vi "GT Pvt Table.vi"(0 "cardNum":i16, 1 "pPos":dbl, 5 "tableId":i16, 7 "count":i32, 9 "pTime":dbl, 11 "error in (no error)":errorcluster caption="错误输入（无错误）", 12 "pVel":dbl) -> (3 "pPos out":dbl, 4 "function return":i16, 10 "pTime out":dbl, 14 "pVel out":dbl, 15 "error out":errorcluster caption="错误输出")   [LabVIEW 2014, in "gts.lvlib"]
doc: "GT_API GT_PvtTable(short cardNum,short tableId,long count,double *pTime,double *pPos,double *pVel);"
uses:
  gts.lvlib
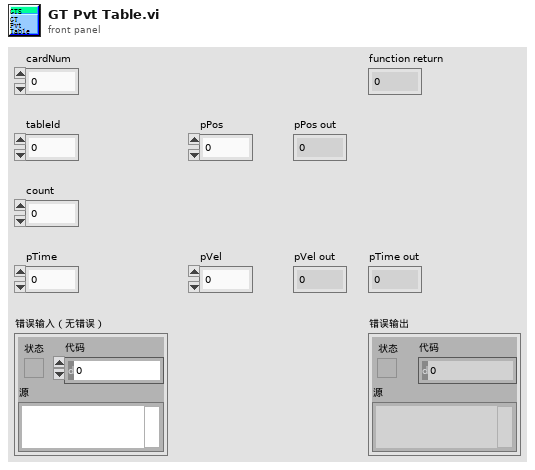
[diagram p1: front panel]
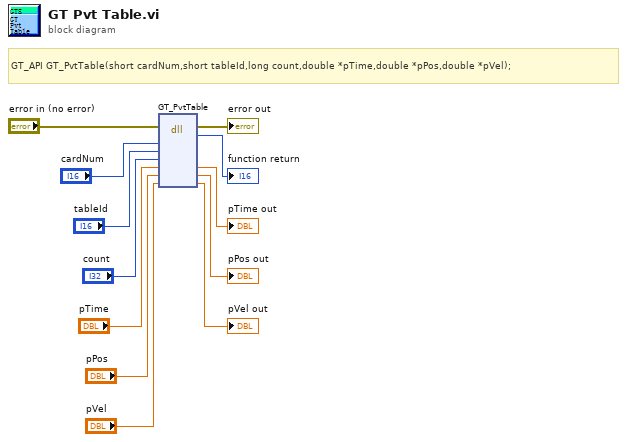
[diagram p0: block diagram]
diagram:
  # "GT_API GT_PvtTable(short cardNum,short tableId,long count,double *pTime,double *pPos,double *pVel);"
  n1 = dll-call lib="PTH2habs D固高科技资料GTS控制卡GTS卡18年上半年资料dllVC32bit\nmulti_cardgts.*" fn="GT_PvtTable"(error in="error in (no error)", "cardNum"="cardNum", "tableId"="tableId", "count"="count", "pTime"="pTime", "pPos"="pPos", "pVel"="pVel") -> (error out=→"error out":errorcluster, →"function return":i16, "pTime"=→"pTime out":dbl, "pPos"=→"pPos out":dbl, "pVel"=→"pVel out":dbl)  [unwired: 5 in, 1 out]
